vi "Shunt - 500 or 10M Control Disable.vi"(8 "error in":errorcluster, 10 "SR":enum16{"500", "10M"}(ring), 11 "reference":refnum<vi>) -> (0 "error out":errorcluster)   [LabVIEW 2016, in "Instrument.KH7008.lvclass"]
uses:
  Instrument.KH7008.lvclass
  typedefs/Shunt-Enum.ctl
panel:
  in  "demo Shunt Resistor":T1=enum."50 Ohms"
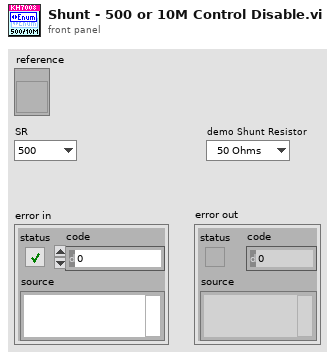
[diagram p1: front panel]
types:
  T1 = typedef "Instrument.KH7008.lvclass/Shunt-Enum.ctl" = enum16{"Open", "50 Ohms", "500 Ohms", "5k Ohms", "50k Ohms", "10M Ohm"}
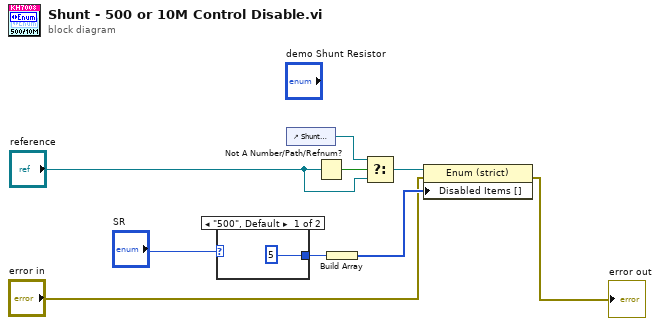
[diagram p0: block diagram]
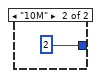
[diagram p2: hidden frame]
diagram:
  n1 = case shown="\"500\", Default" "SR" {
    tunnel: [5 2] -> w9
    frame "500", Default {
    }
    frame "10M" {
    }
  }
  n2 = control-ref of="Shunt Resistor"() -> (w4:refnum<vi>)
  n3 = Not A Number/Path/Refnum?(number/path/refnum="reference") -> (NaN/Path/Refnum?=w7:bool)
  n4 = Build Array(w9) -> (w8:i32[])
  n5 = Select(t=w4, s=w7, f="reference") -> (s? t:f=w6:refnum<vi>)
  n6 = property class="Enum (strict)"(reference=w6, error in="error in", "Disabled Items []"=w8) -> (error out=→"error out":errorcluster)  [unwired: 1 out]
